vi "ATF-Pump-Generate_Event.vi"(8 "error in":errorcluster) -> (0 "error out":errorcluster)   [LabVIEW 2022 SP3]
panel:
  in  "Output level":enum32{"low", "high"}(ring)=enum."high"
  in  "Start Time Delay (Seconds)":ext=5.0
  in  "Output Terminal":tag="/PXI1Slot2/PFI1"
  in  "resource name 2":tag="PXI1Slot2"
  out "Current time":timestamp
  out "Event Time":timestamp format="%<%I:%M:%S%9u %p\n%x>T"
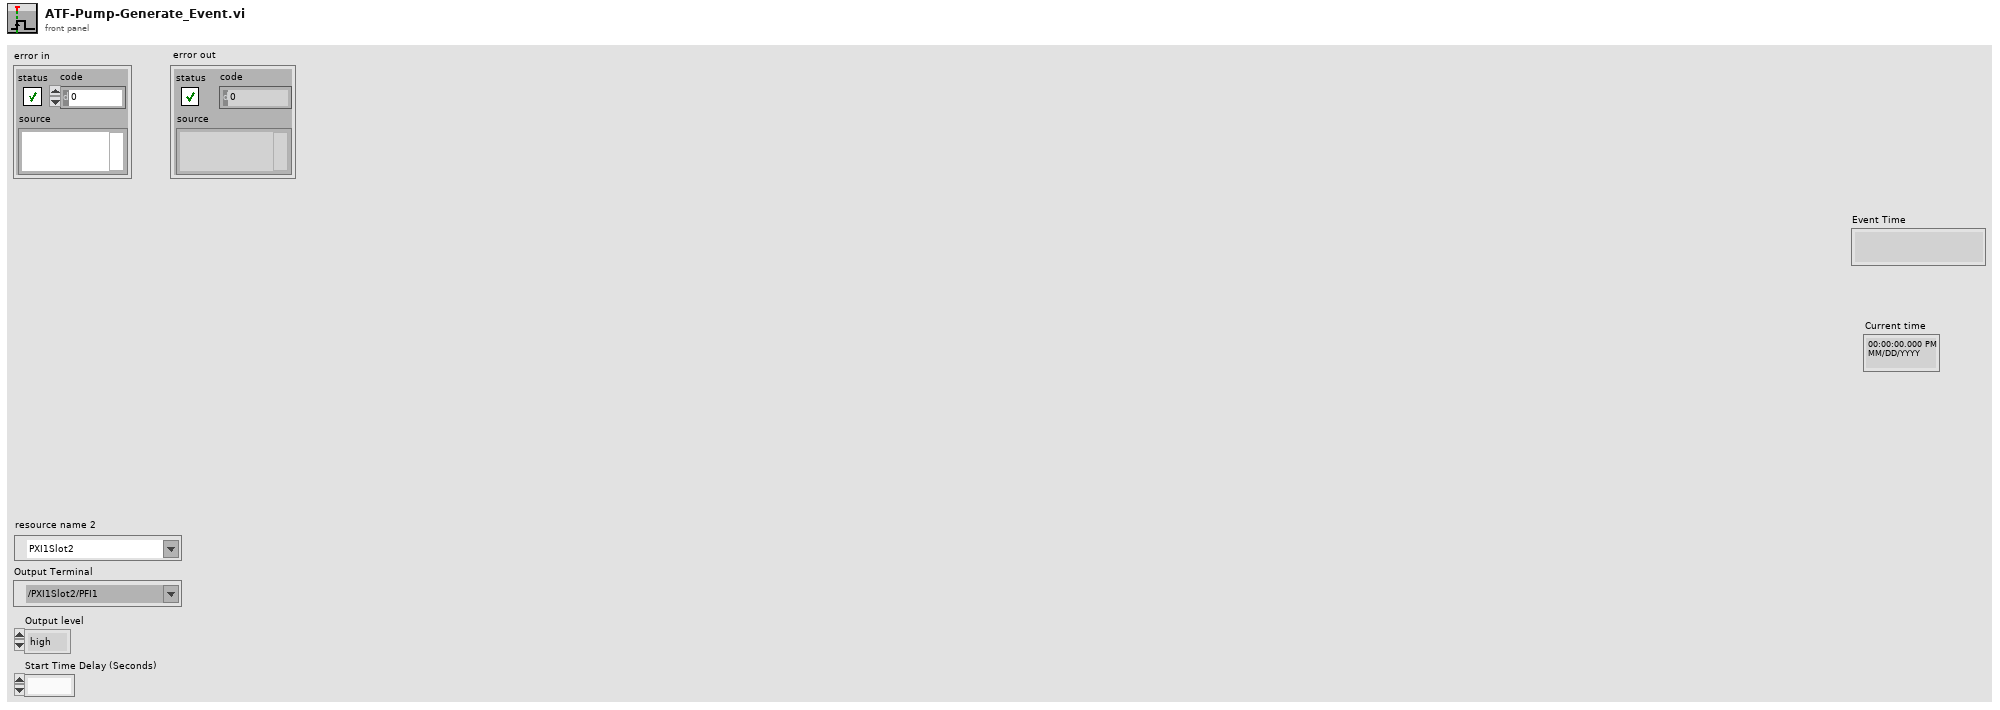
[diagram p1: front panel]
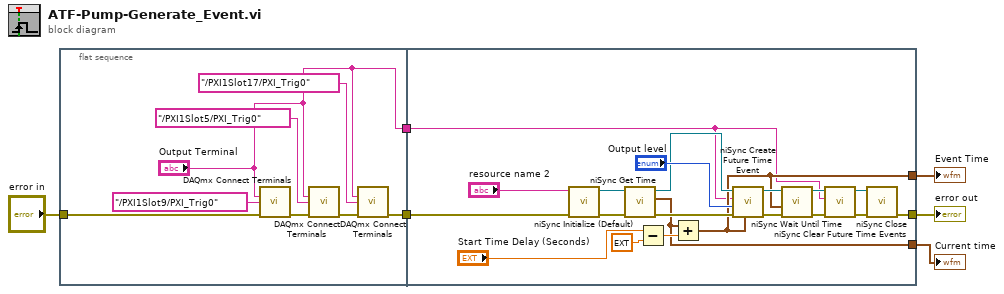
[diagram p0: block diagram]
diagram:
  n1 = flat-sequence {
    tunnel: "error in" -> [w13]
    tunnel: [w7] -> w6
    tunnel: ["Output Terminal"] -> w1
    tunnel: w6 -> [w21]
    tunnel: [w18] -> w4
    tunnel: [w17] -> w3
    tunnel: [w16] -> w2
    tunnel: w1 -> [w15]
    frame #0 {
      n2 = call <vilib>:"DAQmx Connect Terminals.vi"("source terminal"="Output Terminal", "destination terminal"=tag "/PXI1Slot9/PXI_Trig0", "error in"=w13) -> ("error out"=w12:errorcluster)  [unwired: 12 in]
      n3 = call <vilib>:"DAQmx Connect Terminals.vi"("source terminal"="Output Terminal", "destination terminal"=tag "/PXI1Slot5/PXI_Trig0", "error in"=w12) -> ("error out"=w11:errorcluster)  [unwired: 12 in]
      n4 = call <vilib>:"DAQmx Connect Terminals.vi"("source terminal"="Output Terminal", "destination terminal"=tag "/PXI1Slot17/PXI_Trig0", "error in"=w11) -> ("error out"=w7:errorcluster)  [unwired: 12 in]
    }
    frame #1 {
      n5 = call <instrlib>:"niSync Initialize (Default).vi"("error in (no error)"=w21, "resource name"="resource name 2") -> ("error out"=w25:errorcluster, "instrument handle out"=w26:refnum<k15>)  [unwired: 8 in]
      n6 = call <instrlib>:"niSync Get Time.vi"("error in (no error)"=w25, "instrument handle"=w26) -> ("error out"=w31:errorcluster, "time"=w17:timestamp, "instrument handle out"=w32:refnum<k15>)  [unwired: 5 in]
      n7 = Subtract(x="Start Time Delay (Seconds)", y=ext 0.2) -> (x-y=w20:ext)
      n8 = Add(x=w17, y=w20) -> (x+y=w18:timestamp)
      n9 = call <instrlib>:"niSync Create Future Time Event.vi"("time"=w18, "error in (no error)"=w31, "output level"="Output level", "terminal"=w15, "instrument handle"=w32) -> ("error out"=w29:errorcluster, "instrument handle out"=w30:refnum<k15>)  [unwired: 4 in]
      n10 = call <instrlib>:"niSync Wait Until Time.vi"("error in (no error)"=w29, "time stamp"=w18, "instrument handle"=w30) -> ("error out"=w28:errorcluster, "instrument handle out"=w27:refnum<k15>)  [unwired: 3 in]
      n11 = call <instrlib>:"niSync Clear Future Time Events.vi"("error in (no error)"=w28, "terminal"=w15, "instrument handle"=w27) -> ("error out"=w23:errorcluster, "instrument handle out"=w24:refnum<k15>)  [unwired: 6 in]
      n12 = call <instrlib>:"niSync Close.vi"("error in (no error)"=w23, "instrument handle"=w24) -> ("error out"=w16:errorcluster)  [unwired: 9 in]
    }
  }
  "error out" <- w2
  "Event Time" <- w4
  "Current time" <- w3
